vi "Call_exe_py2exe.vi"(8 "error in (no error)":errorcluster caption="entrée d'erreur (pas d'erreur)", 10 "Nom de l'executable":string="Create_Cust_PDF4Box.exe", 11 "Répertoire de travail":path=path "data/pydist") -> (0 "error out":errorcluster)   [LabVIEW 2020]
panel:
  out "chaîne d'entrée":string
  out "Return Code":i32
  out "Standard Error":string
  out "Converted Output":i32
  out "Raw Python String Output":string
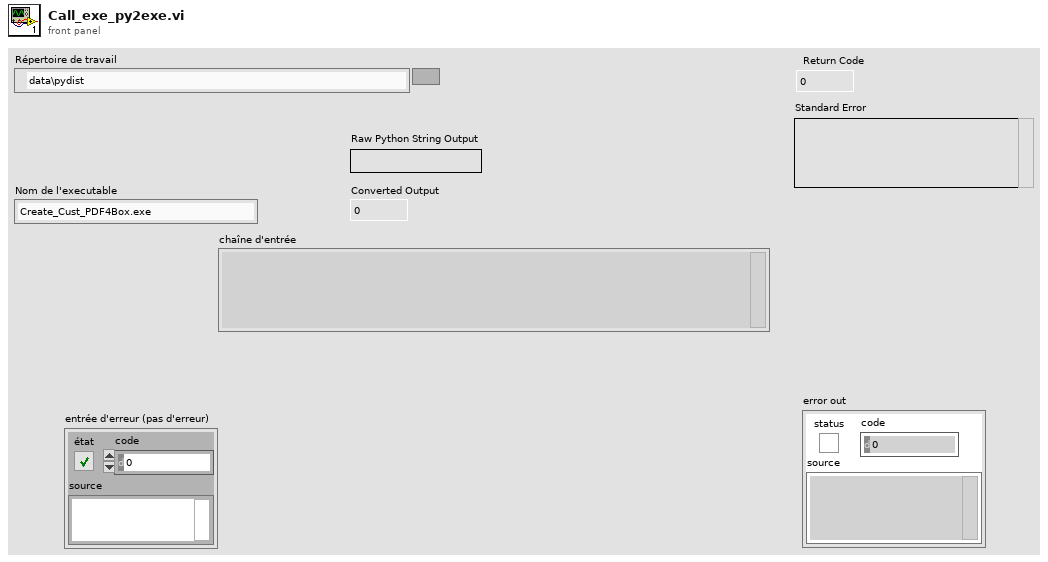
[diagram p1: front panel]
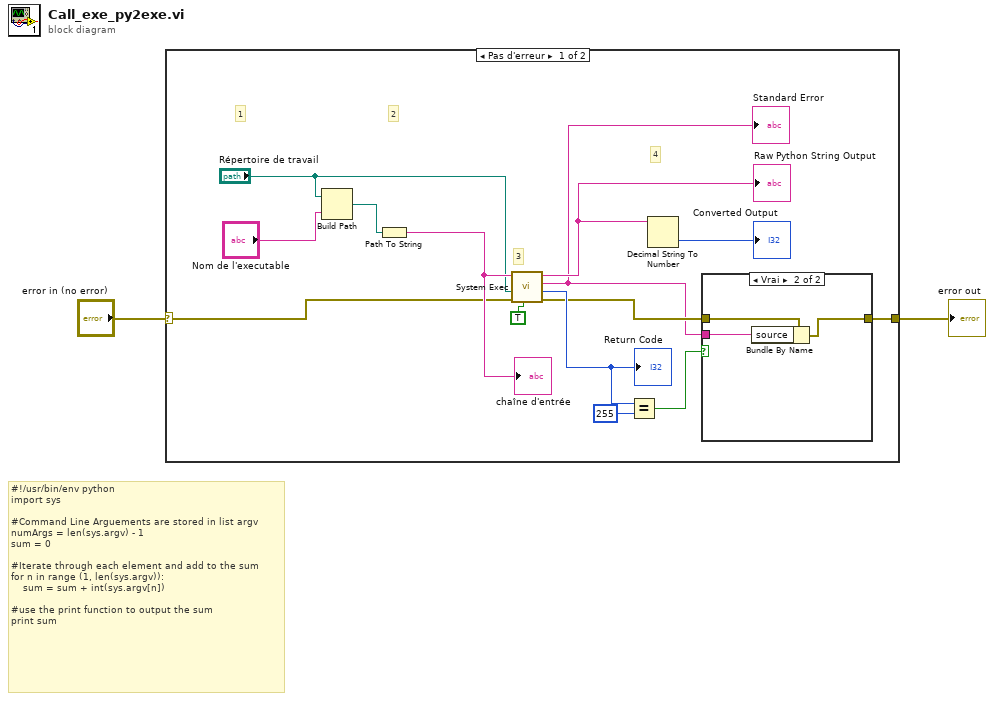
[diagram p0: block diagram]
diagram:
  # "#!/usr/bin/env python\nimport sys\n\n#Command Line Arguements are stored in list argv\nnumArgs = len(sys.argv) - 1\nsum = 0\n\n#Iterate through each element and add to the sum\nfor n in range (1, len(sys.argv)):\n    sum = sum + int(sys.argv[n])\n\n#use the print function to output the sum\nprint sum"
  n1 = case shown="Pas d'erreur" "error in (no error)" {
    selector: "error in (no error)" -> [w10 w21]
    tunnel: [w6 w21] -> w2
    frame No Error {
      # "4"
      # "3"
      # "2"
      # "1"
      n2 = Build Path(base path="Répertoire de travail", name or relative path="Nom de l'executable") -> (appended path=w12:path)
      n3 = Path To String(path=w12) -> (string=w11:string)
      "chaîne d'entrée" <- w11
      n4 = call <vilib>:"System Exec.vi"("run minimized? (F)"=TRUE, "error in (no error)"=w10, "working directory"="Répertoire de travail", "command line"=w11) -> ("error out"=w7:errorcluster, "return code"=w9:i32, "standard error"=w4:string, "standard output"=w15:string)  [unwired: 4 in]
      "Return Code" <- w9
      "Standard Error" <- w4
      "Raw Python String Output" <- w15
      n5 = Equal?(x=w9, y=255) -> (x = y?=w5:bool)
      n6 = Decimal String To Number(string=w15) -> (number=→"Converted Output":i32)  [unwired: 2 in, 1 out]
      n7 = case shown="Vrai" w5 {
        tunnel: w7 -> [w17 w20]
        tunnel: [w17 w19] -> w6
        tunnel: w4 -> [_ w18]
        frame False {
        }
        frame True {
          n8 = Bundle By Name(cluster=w20, "source"=w18) -> (w19:errorcluster)
        }
      }
    }
    frame Error {
    }
  }
  "error out" <- w2
